vi "TX-SIM-BPCS-UDP.vi"() -> ()   [LabVIEW 2017]
uses:
  <vilib>/Platform/TimedLoop/XDataNode/timing_clust.ctl
  <vilib>/Platform/TimedLoop/XDataNode/nitl_modes.ctl
  <vilib>/Platform/TimedLoop/XDataNode/wakeup.ctl
  <vilib>/Platform/TimedLoop/XDataNode/XDataNode.xnode
  <vilib>/Platform/TimedLoop/XDataNode/XDNodeRunTimeDep.lvlib
panel:
  in  "Stop":bool
  out "SIM-BPCS-TX-ARRAY":dbl[](array[numeric])
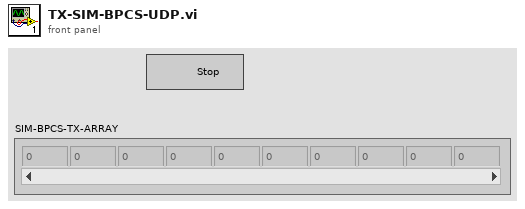
[diagram p1: front panel]
types:
  T1 = typedef "XDNodeRunTimeDep.lvlib/timing_clust.ctl" = cluster{"Expected End [f-1]":u64, "Actual End [f-1]":u64, "Finished Late? [f-1]":bool, "Expected End [i-1]":u64, "Actual End [i-1]":u64, "Finished Late? [i-1]":bool, "Expected Start [i]":u64, "Actual Start [i]":u64, "Expected Start [f]":u64, "Actual Start [f]":u64, "Source Name":string, "Structure Name":string, "Period":i64, "Deadline":i64, "Offset":i64, "Start":i64, "Priority":i32, "Timeout":i32, "Mode":T2, "Wakeup Reason":T3, "Error":errorcluster, "Source Type":string, "Secondary Source Type":string, "Global End Time":u64, "Global Start Time":u64, "Frame Duration":u64, "Iteration Duration":u64, "Assigned CPU":i32, "I/O Scan Engine Mode":u32}
  T2 = typedef "XDNodeRunTimeDep.lvlib/nitl_modes.ctl" = enum32{"No Change", "Process missed periods, maintain original phase", "Discard missed periods, maintain original phase", "Process missed periods, ignore original phase", "Discard missed periods, ignore original phase"}
  T3 = typedef "XDNodeRunTimeDep.lvlib/wakeup.ctl" = enum32{"Normal", "Aborted", "Asynchronous wakeup", "Timing source error", "Timed loop error", "Timeout"}
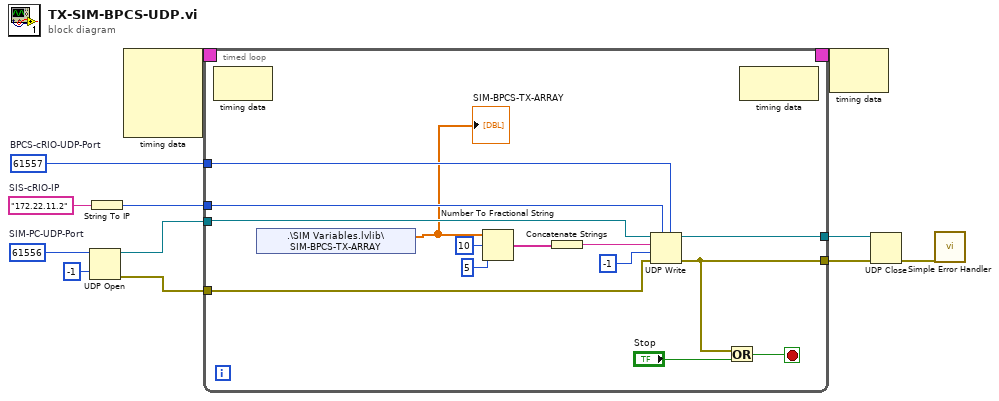
[diagram p0: block diagram]
diagram:
  w7 = u16 61556  # SIM-PC-UDP-Port
  w8 = u16 61557  # BPCS-cRIO-UDP-Port
  w10 = "172.22.11.2"  # SIS-cRIO-IP
  n1 = UDP Open(9:-1 ("timeout ms (25000)"), 11:w7) -> (port=w6:refnum<k16>, 0:w5:errorcluster)  [unwired: 3 in, 1 out]
  n2 = String To IP(1:w10) -> (0:w9:u32)
  n3 = node-c288() -> (w12:T1)  [unwired: 4 in]
  n4 = timed-loop {
    timing: w12 -> [_]
    timing-out: [_] -> w11
    tunnel: w9 -> [w25]
    tunnel: w8 -> [w24]
    tunnel: w6 -> [w23]
    tunnel: w5 -> [w22]
    tunnel: [w21] -> w4
    tunnel: [w20] -> w3
    stop <- w18 stop-if-true
    n5 = node-c288() -> ()  [unwired: 1 in, 1 out]
    n6 = shared-variable ".\\SIM Variables.lvlib\\SIM-BPCS-TX-ARRAY"() -> (w14:dbl[])  [unwired: 1 in, 1 out]
    "SIM-BPCS-TX-ARRAY" <- w14
    n7 = Number To Fractional String(number=w14, width (-)=i16 10, precision (6)=i16 5) -> (F-format string=w17:string[])  [unwired: 1 in]
    n8 = Concatenate Strings(w17) -> (w26:string)
    n9 = UDP Write(address=w25, port or service name=w24, connection ID=w23, data in=w26, 8:w22, 9:-1 ("timeout ms (25000)")) -> (error out=w20:errorcluster, 3:w21:refnum<k16>)
    n10 = Or(x=w20, y="Stop") -> (x .or. y?=w18:bool)
    n11 = node-c288() -> ()  [unwired: 1 in, 1 out]
  }
  n12 = node-c288(w11) -> ()  [unwired: 1 out]
  n13 = UDP Close(connection ID=w4, 8:w3) -> (error out=w2:errorcluster)  [unwired: 1 out]
  n14 = call <vilib>:"Simple Error Handler.vi"("error in (no error)"=w2) -> ()  [unwired: 4 in, 5 out]
